vi "Test Magnet.vi"(8 "error in (no error)":errorcluster, 11 "Instrument.Cryostat in":refnum<class "Instrument.Cryostat.lvclass">) -> (0 "error out":errorcluster, 3 "Instrument.Cryostat out":refnum<class "Instrument.Cryostat.lvclass">)   [LabVIEW 2016, in "Instrument.Cryostat.lvclass"]
uses:
  Instrument.Cryostat.lvclass
  <vilib>/addons/_JKI Toolkits/Caraya/classes/Assert/Assert.lvclass
  <vilib>/addons/_JKI Toolkits/Caraya/classes/Test/Test.lvclass
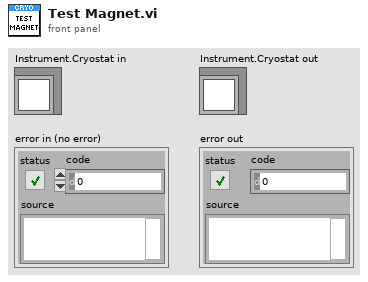
[diagram p1: front panel]
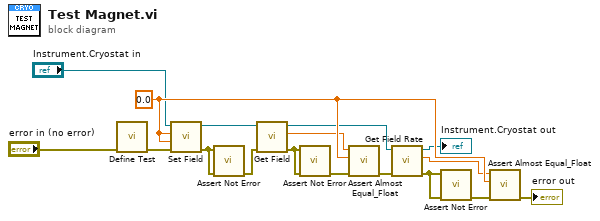
[diagram p0: block diagram]
diagram:
  w9 = 0.0 ("Angle (°)")
  n1 = call <vilib>:"Define Test.vi"("error in (no error)"="error in (no error)") -> ("error out"=w1:errorcluster)  [unwired: 10 in]
  n2 = call-dynamic "Set Field.vi"("error in (no error)"=w1, "Rate (T/min)"=w9, "Field (T)"=w9, "Instrument.Cryostat in"="Instrument.Cryostat in") -> ("error out"=w10:errorcluster, "Instrument.Cryostat out"=w6:refnum<class "Instrument.Cryostat.lvclass">)  [unwired: 6 in]
  n3 = call <vilib>:"Assert Not Error.vi"("error in (no error)"=w10, "Not Error?"=w10) -> ("error out"=w11:errorcluster)  [unwired: 9 in]
  n4 = call-dynamic "Get Field.vi"("error in (no error)"=w11, "Instrument.Cryostat in"=w6) -> ("error out"=w12:errorcluster, "B Field (T)"=w3:dbl, "Instrument.Cryostat out"=w5:refnum<class "Instrument.Cryostat.lvclass">)  [unwired: 7 in]
  n5 = call <vilib>:"Assert Not Error.vi"("error in (no error)"=w12, "Not Error?"=w12) -> ("error out"=w13:errorcluster)  [unwired: 9 in]
  n6 = call <vilib>:"Assert Almost Equal_Float.vi"("error in (no error)"=w13, "Y"=w9, "X"=w3) -> ("error out"=w14:errorcluster)  [unwired: 8 in]
  n7 = call-dynamic "Get Field Rate.vi"("error in (no error)"=w14, "Instrument.Cryostat in"=w5) -> ("error out"=w15:errorcluster, "B Field Rate (T/min)"=w4:dbl, "Instrument.Cryostat out"=→"Instrument.Cryostat out":refnum<class "Instrument.Cryostat.lvclass">)  [unwired: 7 in]
  n8 = call <vilib>:"Assert Not Error.vi"("error in (no error)"=w15, "Not Error?"=w15) -> ("error out"=w16:errorcluster)  [unwired: 9 in]
  n9 = call <vilib>:"Assert Almost Equal_Float.vi"("error in (no error)"=w16, "Y"=w9, "X"=w4) -> ("error out"=→"error out":errorcluster)  [unwired: 8 in]
